vi "Subscribe (SingleTopic).vi"(6 "timeout (100ms)":i32=100, 8 "error in (no error)":errorcluster, 9 "QoS":T1, 10 "Topic Filter":string, 11 "MQTT_Base in":refnum<class "MQTT_Base.lvclass">) -> (0 "error out":errorcluster, 3 "MQTT_Base out":refnum<class "MQTT_Base.lvclass">)   [LabVIEW 2013, in "MQTT Base.lvlib" / "MQTT_Base.lvclass"]
uses:
  MQTT_Base.lvclass
  <vilib>/LabVIEW Open Source Project/MQTT Control Packets/Control Packets/ControlPacket/QualityOfService -- enum.ctl
  <vilib>/LabVIEW Open Source Project/MQTT Control Packets/Control Packets/SUBSCRIBE/Topic Subscription -- cluster.ctl
  <vilib>/LabVIEW Open Source Project/MQTT Control Packets/Control Packets/SUBSCRIBE/SUBSCRIBE.lvclass
  <vilib>/LabVIEW Open Source Project/MQTT Control Packets/Control Packets/ControlPacket/ControlPacket.lvclass
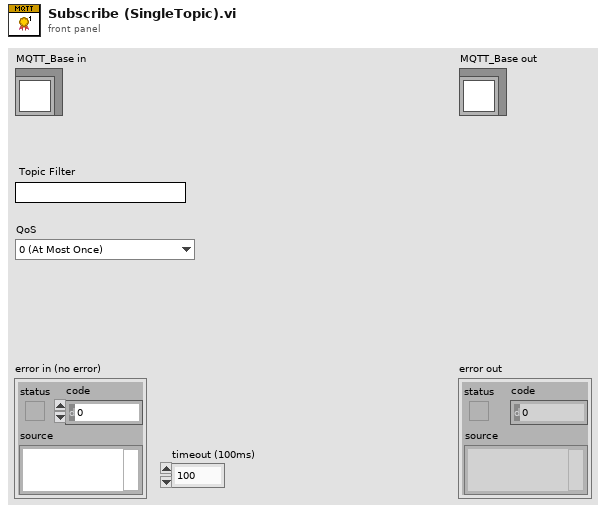
[diagram p1: front panel]
types:
  T1 = typedef "MQTT_Control_Packets.lvlib/ControlPacket.lvclass/QualityOfService -- enum.ctl" = enum16{"0 (At Most Once)", "1 (At Least Once)", "2 (Exactly Once)"}
  T2 = typedef "MQTT_Control_Packets.lvlib/SUBSCRIBE.lvclass/Topic Subscription -- cluster.ctl" = cluster{"Topic Filter":string, "QoS":T1}
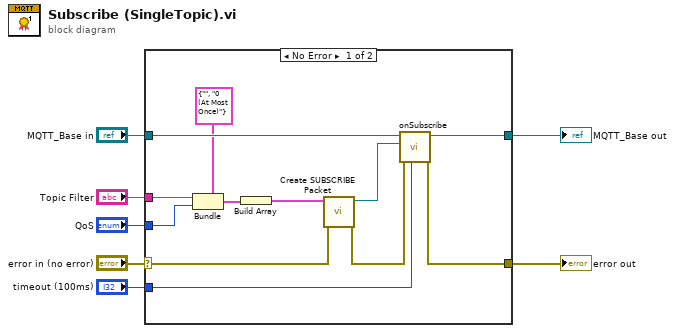
[diagram p0: block diagram]
diagram:
  n1 = case shown="No Error" "error in (no error)" {
    selector: "error in (no error)" -> [w14 w21]
    tunnel: [w17 w21] -> w6
    tunnel: [w18 w20] -> w4
    tunnel: "MQTT_Base in" -> [w19 w20]
    tunnel: "Topic Filter" -> [w13 _]
    tunnel: "QoS" -> [w12 _]
    tunnel: "timeout (100ms)" -> [w8 _]
    frame No Error {
      n2 = Bundle(cluster=T2 {"Topic Filter"="", "QoS"=enum."0 (At Most Once)"} ("Topic Subscription"), "Topic Filter"=w13, "QoS"=w12) -> (w11:T2)
      n3 = Build Array(w11) -> (w10:T2[])
      n4 = call <vilib>:"Create SUBSCRIBE Packet.vi"("error in (no error)"=w14, "Topic Subscriptions"=w10) -> ("error out"=w15:errorcluster, "SUBSCRIBE out"=w16:refnum<class "SUBSCRIBE.lvclass">)  [unwired: 7 in, 1 out]
      n5 = call-dynamic "onSubscribe.vi"("timeout (100ms)"=w8, "error in (no error)"=w15, "SUBSCRIBE"=w16, "MQTT_Base in"=w19) -> ("error out"=w17:errorcluster, "MQTT_Base out"=w18:refnum<class "MQTT_Base.lvclass">)  [unwired: 5 in, 1 out]
    }
    frame Error {
    }
  }
  "error out" <- w6
  "MQTT_Base out" <- w4
